vi "Build.vi"(0 "NSIS Installer In":refnum<class "NSIS Installer.lvclass">) -> (4 "NSIS Installer Out":refnum<class "NSIS Installer.lvclass">)   [LabVIEW 2017, in "CL_G3_VIComponentBuilder.lvlib" / "NSIS Installer.lvclass"]
doc: "Creates the installer."
uses:
  NSIS Installer.lvclass
  C:/Tool Chain Support/Software Module Builder/Source/Exports/Exports/Export.lvclass
  Exports/Export.lvclass/Export.ctl
  Exports/Accessors/Read Component Export Dir.vi
  Exports/Accessors/Read Export Build Specification.vi
  Exports/Accessors/Write Exported Build Specification Path.vi
  Exports/Accessors/Write Export Operation Errors.vi
  Exports/Accessors/Read Export Operation Errors.vi
  Compound Installer/Compound_Installer.lvclass
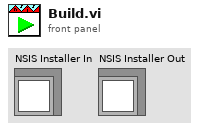
[diagram p1: front panel]
types:
  T1 = cluster{"Compound_Installer":refnum<class "NSIS Installer.lvclass">}
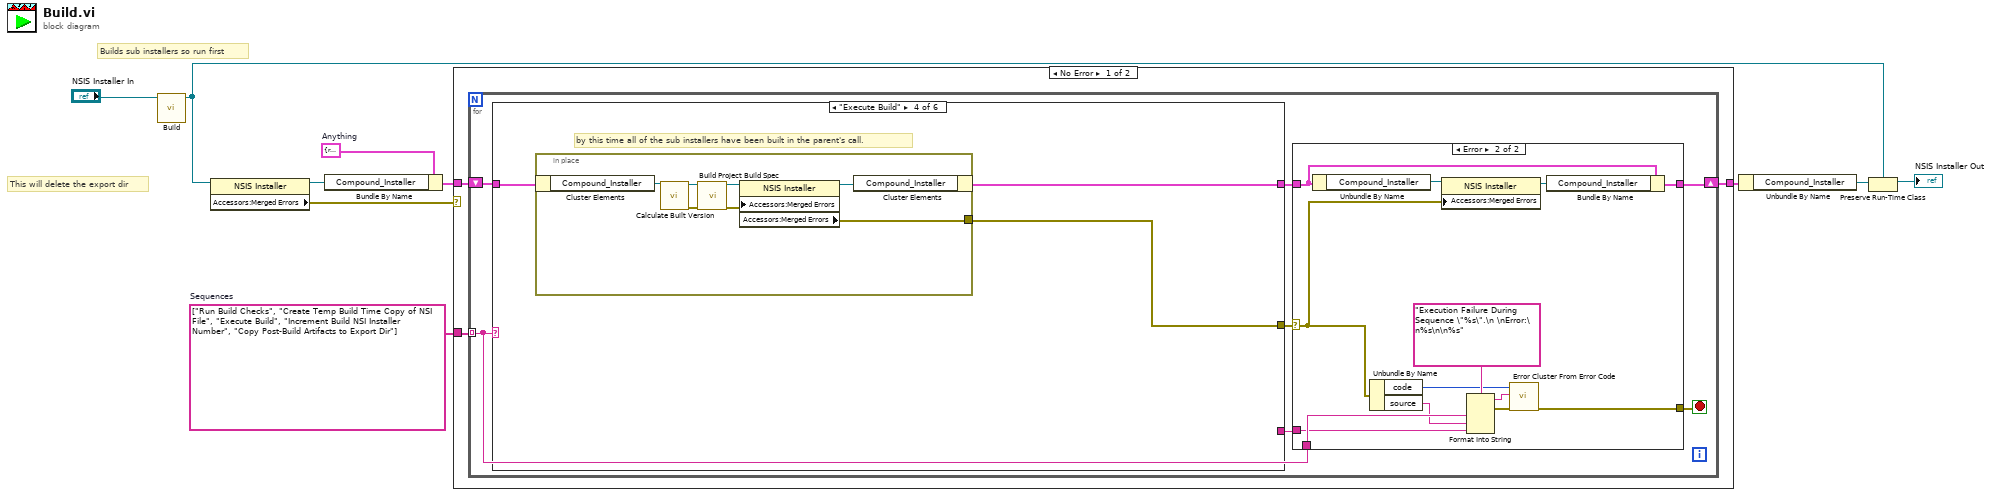
[diagram p0: block diagram]
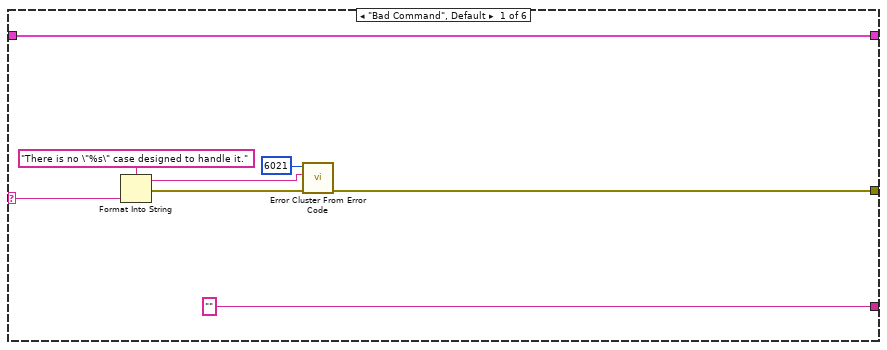
[diagram p3: hidden frame]
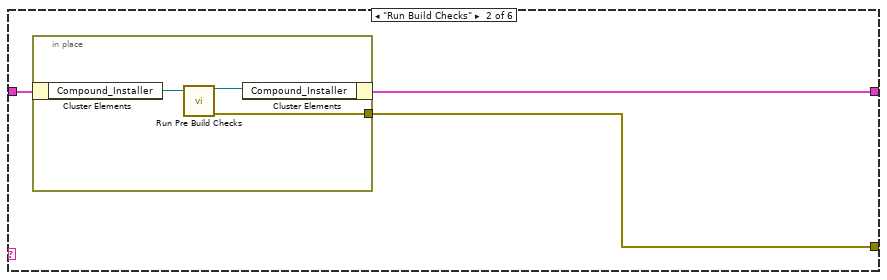
[diagram p4: hidden frame]
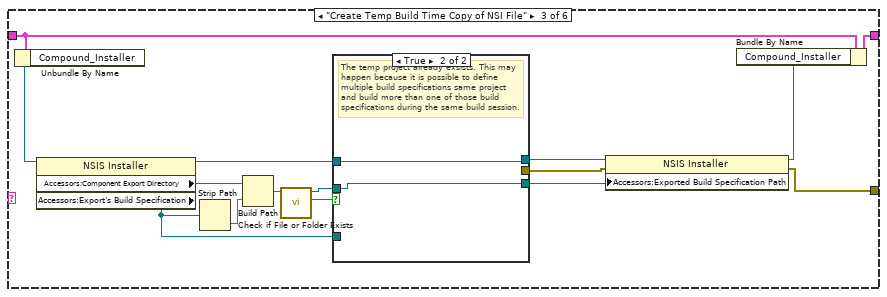
[diagram p5: hidden frame]
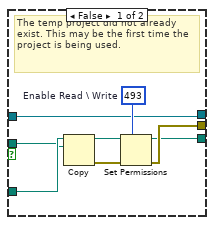
[diagram p6: hidden frame]
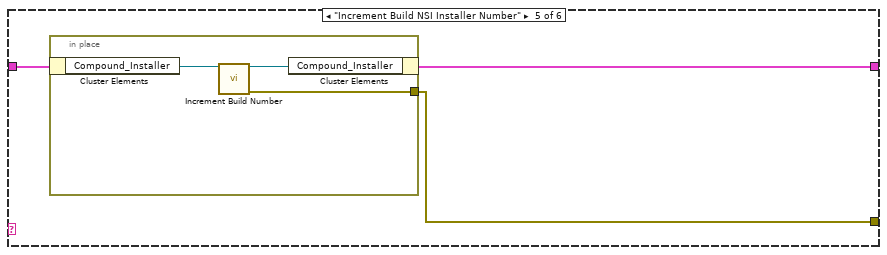
[diagram p7: hidden frame]
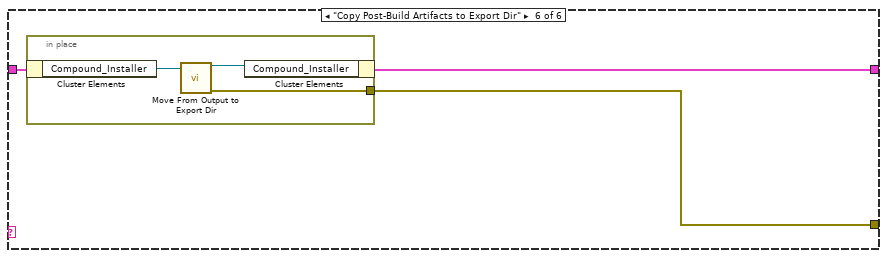
[diagram p8: hidden frame]
diagram:
  w7 = T1 {"Compound_Installer"=refnum}  # Anything
  w9 = string[] ["Run Build Checks", "Create Temp Build Time Copy of NSI File", "Execute Build", "Increment Build NSI Installer Number", "Copy Post-Build Artifacts to Export Dir"]  # Sequences
  # "This will delete the export dir"
  # "Builds sub installers so run first"
  n1 = call-parent "Build.vi"("Compound_Installer In"="NSIS Installer In") -> ("Compound_Installer Out"=w5:refnum<class "NSIS Installer.lvclass">)  [unwired: 14 in]
  n2 = property class="NSIS Installer"(reference=w5) -> (reference out=w3:refnum<class "NSIS Installer.lvclass">, "Accessors:Merged Errors"=w2:errorcluster)  [unwired: 1 in, 1 out]
  n3 = Bundle By Name(cluster=w7, "Compound_Installer"=w3) -> (w10:T1)
  n4 = case shown="No Error" w2 {
    tunnel: w9 -> [w13 _]
    tunnel: w10 -> [w12 w97]
    tunnel: [w11 w97] -> w8
    frame No Error {
      n5 = for {
        tunnel: w13 -> [w19] mode=indexing
        shift-right: [w15] -> w11
        shift-left: w12 -> [w20]
        stop <- w17 stop-if-true
        n6 = case shown="\"Execute Build\"" w19 {
          selector: w19 -> [w40 _ _ _ _ _]
          tunnel: w20 -> [w43 w46 w64 w76 w87 w93]
          tunnel: [w43 w44 w57 w75 w86 w91] -> w16
          tunnel: [w39 w45 w55 w77 w85 w92] -> w14
          tunnel: ["" ("Accessors:Name") _ _ _ _ _] -> w18
          frame "Bad Command", Default {
            n7 = Format Into String(format string="There is no \"%s\" case designed to handle it.", w40) -> (resulting string=w38:string, error out=w36:errorcluster)  [unwired: 2 in]
            n8 = call <vilib>:"Error Cluster From Error Code.vi"("error in (no error)"=w36, "error message (\"\")"=w38, "error code (0)"=6021 ("Error Code")) -> ("error out"=w39:errorcluster)  [unwired: 6 in]
          }
          frame "Run Build Checks" {
            n9 = in-place {
              in-place-border: [w47] -> w45
              n10 = in-place-cluster #1(w46) -> ("Compound_Installer"=w49:refnum<class "NSIS Installer.lvclass">)
              n11 = call-dynamic "Run Pre Build Checks.vi"("NSIS Installer"=w49) -> ("NSIS Installer"=w48:refnum<class "NSIS Installer.lvclass">, "error out"=w47:errorcluster)  [unwired: 13 in]
              n12 = in-place-cluster #1("Compound_Installer"=w48) -> (w44:T1)
            }
          }
          frame "Create Temp Build Time Copy of NSI File" {
            n13 = Unbundle By Name(w64) -> ("Compound_Installer"=w58:refnum<class "NSIS Installer.lvclass">)
            n14 = property class="NSIS Installer"(reference=w58) -> (reference out=w63:refnum<class "NSIS Installer.lvclass">, "Accessors:Component Export Directory"=w54:path, "Accessors:Export's Build Specification"=w51:path)  [unwired: 1 in, 1 out]
            n15 = Strip Path(path=w51) -> (name=w53:string)  [unwired: 1 out]
            n16 = Build Path(base path=w54, name or relative path=w53) -> (appended path=w52:path)
            n17 = call <vilib>:"Check if File or Folder Exists.vi"("path"=w52) -> ("file or folder exists?"=w59:bool, "dup path"=w50:path)  [unwired: 8 in, 1 out]
            n18 = case shown="True" w59 {
              tunnel: w63 -> [w67 w74]
              tunnel: [w67 w74] -> w60
              tunnel: [w69 _] -> w61
              tunnel: [w68 w73] -> w62
              tunnel: w51 -> [w66 _]
              tunnel: w50 -> [w65 w73]
              frame False {
                w70 = i16 493  # Enable Read \ Write
                # "The temp project did not already exist. This may be the first time the project is being used."
                n19 = Copy(10:w65, 11:w66) -> (0:w71:errorcluster, 3:w72:path)  [unwired: 3 in, 1 out]
                n20 = Set Permissions(7:w70, 8:w71, 11:w72) -> (0:w69:errorcluster, 3:w68:path)  [unwired: 2 in]
              }
              frame True {
                # "The temp project already exsists. This may happen because it is possible to define multiple build specifications same project and build more than one of those build specifications during the same build session."
              }
            }
            n21 = property class="NSIS Installer"(reference=w60, error in=w61, "Accessors:Exported Build Specification Path"=w62) -> (reference out=w56:refnum<class "NSIS Installer.lvclass">, error out=w55:errorcluster)
            n22 = Bundle By Name(cluster=w64, "Compound_Installer"=w56) -> (w57:T1)
          }
          frame "Execute Build" {
            # "by this time all of the sub installers have been built in the parent's call."
            n23 = in-place {
              in-place-border: [w84] -> w77
              n24 = in-place-cluster #2(w76) -> ("Compound_Installer"=w80:refnum<class "NSIS Installer.lvclass">)
              n25 = call-dynamic "Calculate Built Version.vi"("Export in"=w80) -> ("Export out"=w79:refnum<class "NSIS Installer.lvclass">, "error out"=w78:errorcluster)  [unwired: 13 in]
              n26 = call-dynamic "Build Project Build Spec.vi"("NSIS Installer"=w79, "error IO"=w78) -> ("NSIS Installer"=w83:refnum<class "NSIS Installer.lvclass">, "error out"=w82:errorcluster)  [unwired: 12 in]
              n27 = property class="NSIS Installer"(reference=w83, "Accessors:Merged Errors"=w82) -> (reference out=w81:refnum<class "NSIS Installer.lvclass">, "Accessors:Merged Errors"=w84:errorcluster)  [unwired: 1 in, 1 out]
              n28 = in-place-cluster #2("Compound_Installer"=w81) -> (w75:T1)
            }
          }
          frame "Increment Build NSI Installer Number" {
            n29 = in-place {
              in-place-border: [w90] -> w85
              n30 = in-place-cluster #3(w87) -> ("Compound_Installer"=w89:refnum<class "NSIS Installer.lvclass">)
              n31 = call-dynamic "Increment Build Number.vi"("Compound_Installer in"=w89) -> ("Compound_Installer out"=w88:refnum<class "NSIS Installer.lvclass">, "error out"=w90:errorcluster)  [unwired: 13 in]
              n32 = in-place-cluster #3("Compound_Installer"=w88) -> (w86:T1)
            }
          }
          frame "Copy Post-Build Artifacts to Export Dir" {
            n33 = in-place {
              in-place-border: [w94] -> w92
              n34 = in-place-cluster #4(w93) -> ("Compound_Installer"=w96:refnum<class "NSIS Installer.lvclass">)
              n35 = call-dynamic "Move From Output to Export Dir.vi"("CL_G3_VIComponentBuilder.lvlib:Compound_Installer"=w96) -> ("CL_G3_VIComponentBuilder.lvlib:Compound_Installer"=w95:refnum<class "NSIS Installer.lvclass">, "error out"=w94:errorcluster)  [unwired: 13 in]
              n36 = in-place-cluster #4("Compound_Installer"=w95) -> (w91:T1)
            }
          }
        }
        n37 = case shown="Error" w14 {
          selector: w14 -> [w22 w26]
          tunnel: [w22 w35] -> w17
          tunnel: w19 -> [_ w33]
          tunnel: w18 -> [_ w30]
          tunnel: w16 -> [w21 w25]
          tunnel: [w21 w23] -> w15
          frame No Error {
          }
          frame Error {
            n38 = Unbundle By Name(w25) -> ("Compound_Installer"=w27:refnum<class "NSIS Installer.lvclass">)
            n39 = Unbundle By Name(w26) -> ("code"=w28:i32, "source"=w31:string)
            n40 = property class="NSIS Installer"(reference=w27, "Accessors:Merged Errors"=w26) -> (reference out=w24:refnum<class "NSIS Installer.lvclass">)  [unwired: 1 in, 1 out]
            n41 = Format Into String(format string="Execution Failure During Sequence \"%s\".\n \nError:\n%s\n\n%s" ("error message (\"\")"), w33, w31, w30) -> (resulting string=w34:string, error out=w29:errorcluster)  [unwired: 2 in]
            n42 = call <vilib>:"Error Cluster From Error Code.vi"("error in (no error)"=w29, "error message (\"\")"=w34, "error code (0)"=w28) -> ("error out"=w35:errorcluster)  [unwired: 6 in]
            n43 = Bundle By Name(cluster=w25, "Compound_Installer"=w24) -> (w23:T1)
          }
        }
      }
    }
    frame Error {
    }
  }
  n44 = Unbundle By Name(w8) -> ("Compound_Installer"=w4:refnum<class "NSIS Installer.lvclass">)
  n45 = Preserve Run-Time Class(object in=w4, 2:w5) -> (object out=→"NSIS Installer Out":refnum<class "NSIS Installer.lvclass">)  [unwired: 1 in, 1 out]
